vi "Save_Value_in_Track_Displ_Array-1.vi"(3 "[IN] Value":dbl, 4 "[IN] Index":i32, 5 "[IN] Empty tracks\nfor points saving":dbl[](array[numeric])) -> (1 "[OUT] Index ++":i32, 2 "[OUT Track with saved value":dbl[](array[numeric]))   [LabVIEW 2017]
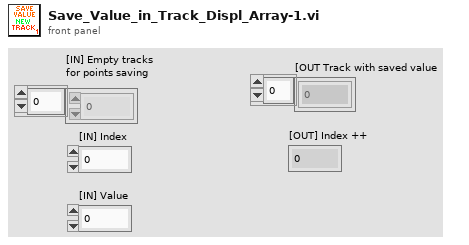
[diagram p1: front panel]
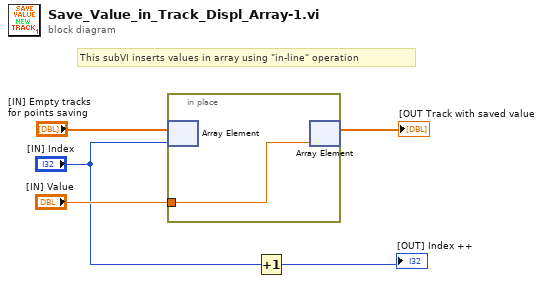
[diagram p0: block diagram]
diagram:
  # "This subVI inserts values in array using \"in-line\" operation"
  n1 = in-place {
    in-place-border: "[IN] Value" -> [w6]
    n2 = in-place-array #1("[IN] Empty tracks\nfor points saving", "[IN] Index") -> ()  [unwired: 1 out]
    n3 = in-place-array #1(w6) -> (→"[OUT Track with saved value":dbl[])  [unwired: 1 out]
  }
  n4 = Increment(x="[IN] Index") -> (x+1=→"[OUT] Index ++":i32)
